vi "CRYSet Channel State.vi"(4 "New Channel Info":T1[](array[typedef]) {"Coupling" items=["Default"=-1, "RSE"=10083, "NRSE"=10078, "Differential"=10106, "Pseudodifferential"=12529]; "term config" items=["Default"=-1, "RSE"=10083, "NRSE"=10078, "Differential"=10106, "Pseudodifferential"=12529]; "Anti-aliasing Factor (%fs)" format="%.2f"}, 6 "Old Channel Info":T1[](array[typedef]) {"Coupling" items=["Default"=-1, "RSE"=10083, "NRSE"=10078, "Differential"=10106, "Pseudodifferential"=12529]; "term config" items=["Default"=-1, "RSE"=10083, "NRSE"=10078, "Differential"=10106, "Pseudodifferential"=12529]; "Anti-aliasing Factor (%fs)" format="%.2f"}, 9 "New Name In":string[][](array[string]), 10 "Old Name In":string[][](array[string]), 11 "Mode":enum16{"Load", "SaveAs", "Revert"}(ring)) -> (0 "Name Out":string[][](array[string]))   [LabVIEW 2013]
uses:
  Typedef Control/CRYHardware Channel Info.ctl
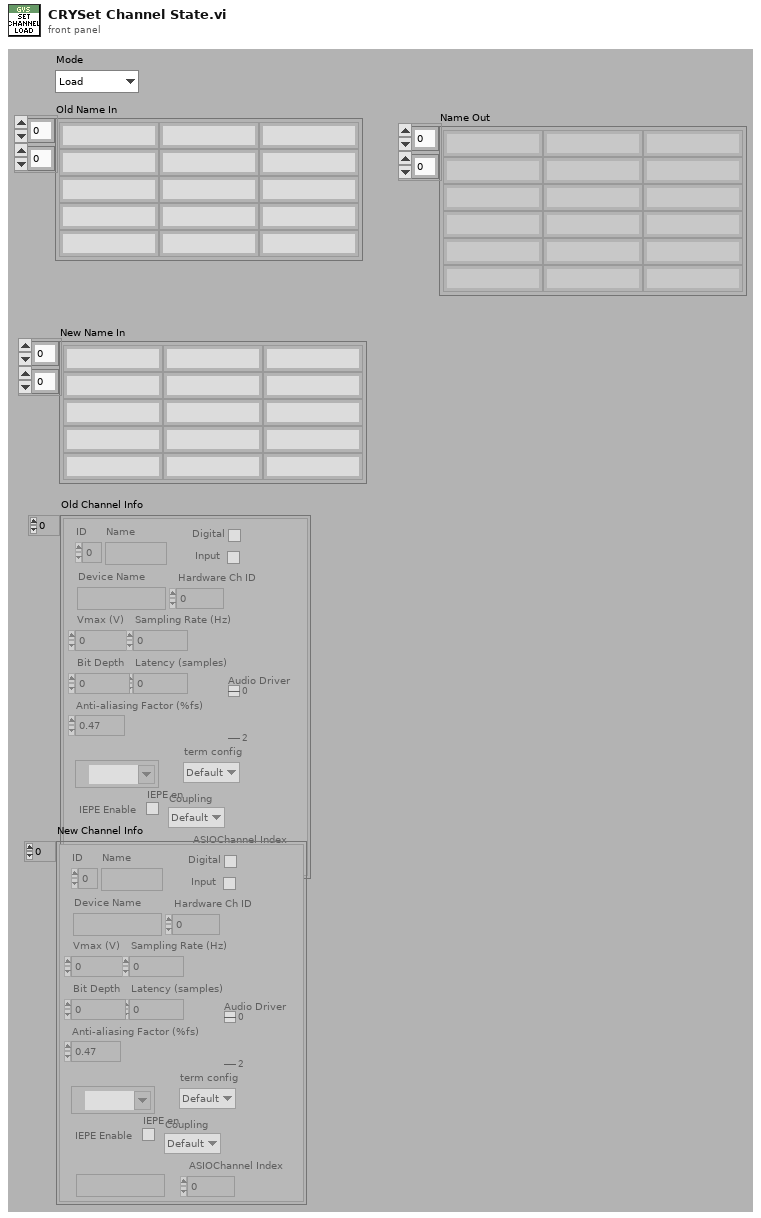
[diagram p1: front panel]
types:
  T1 = typedef "CRYHardware Channel Info.ctl" = cluster{"ID":i32, "Name":string, "Digital":bool, "Input":bool, "Device Name":string, "Hardware Ch ID":u8, "Vmax (V)":dbl, "Latency (samples)":dbl, "Sampling Rate (Hz)":u32, "Bit Depth":u32, "Anti-aliasing Factor (%fs)":sgl, "DAQmx Channel":tag, "term config":i32, "Coupling":i32, "IEPE en":bool, "ASIOChannel Name":string, "Audio Driver":u16, "ASIOChannel Index":u8}
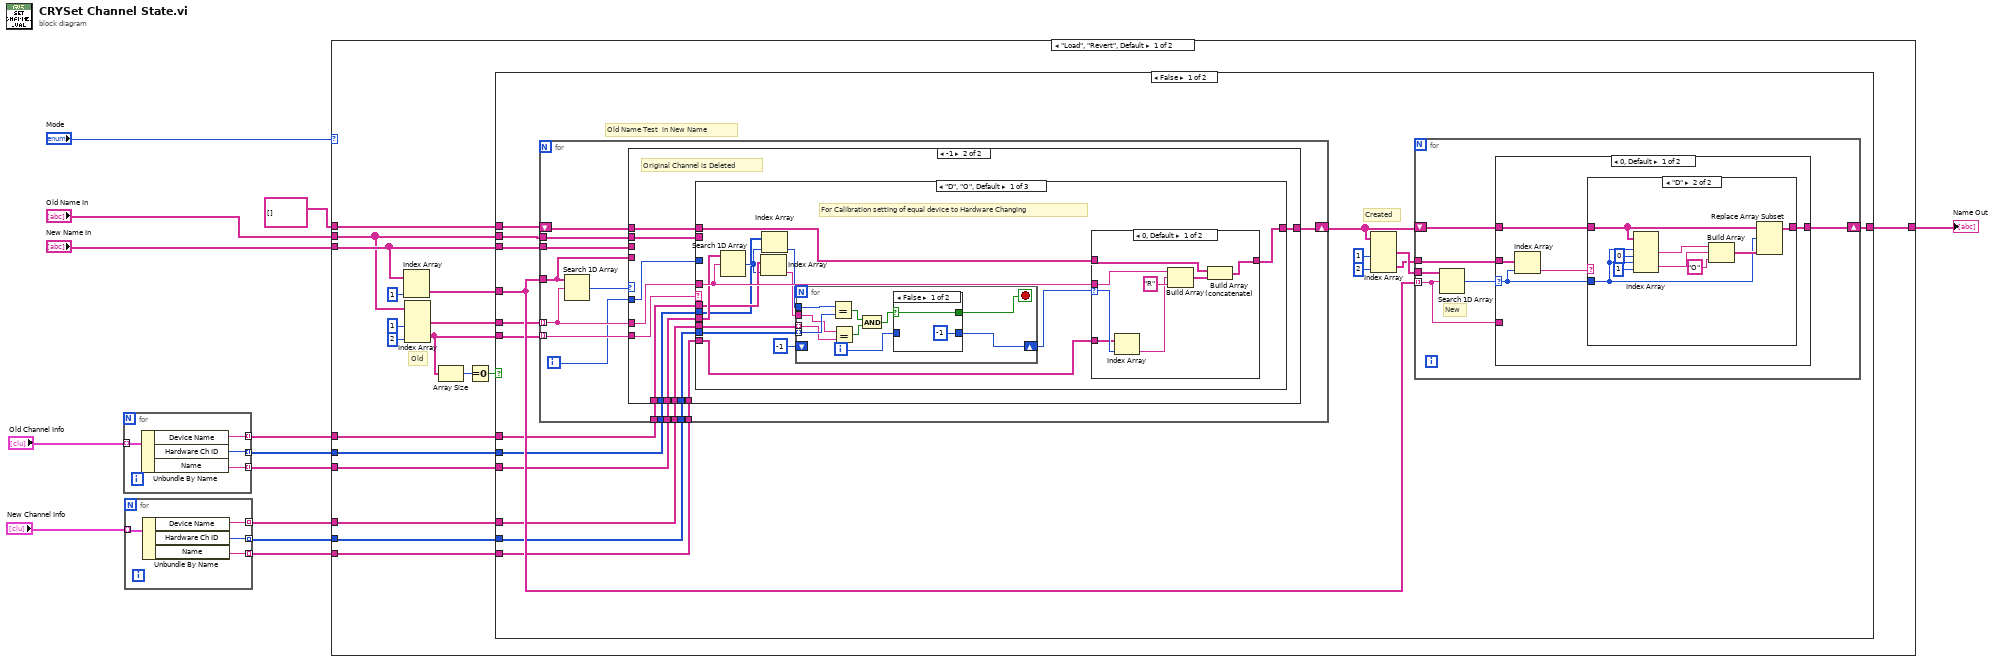
[diagram p0: block diagram]
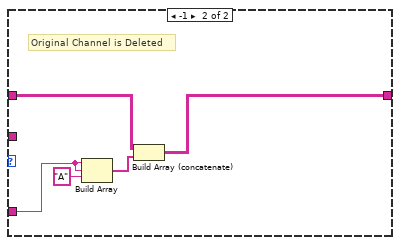
[diagram p3: hidden frame]
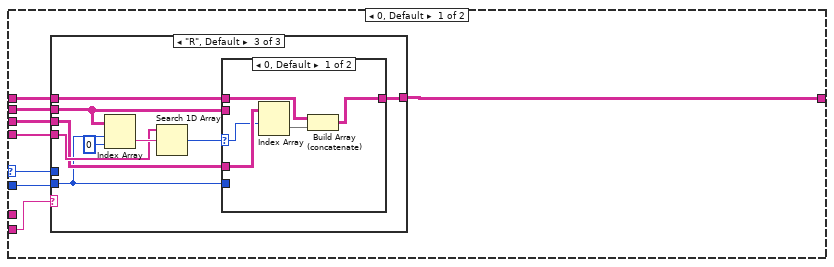
[diagram p4: hidden frame]
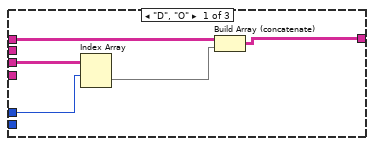
[diagram p5: hidden frame]
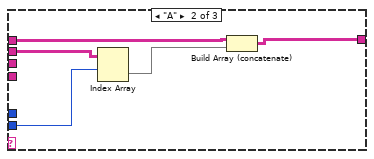
[diagram p6: hidden frame]
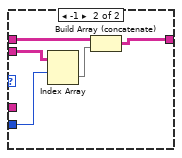
[diagram p7: hidden frame]
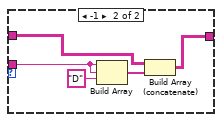
[diagram p9: hidden frame]
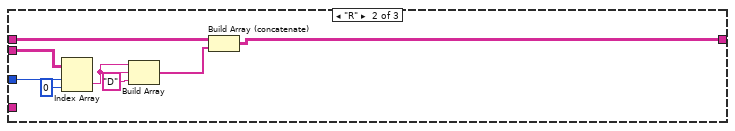
[diagram p10: hidden frame]
diagram:
  n1 = for {
    tunnel: "Old Channel Info" -> [w17] mode=indexing
    tunnel: [w16] -> w8 mode=indexing
    tunnel: [w15] -> w7 mode=indexing
    tunnel: [w14] -> w3 mode=indexing
    n2 = Unbundle By Name(w17) -> ("Device Name"=w16:string, "Hardware Ch ID"=w15:u8, "Name"=w14:string)
  }
  n3 = for {
    tunnel: "New Channel Info" -> [w21] mode=indexing
    tunnel: [w20] -> w5 mode=indexing
    tunnel: [w19] -> w4 mode=indexing
    tunnel: [w18] -> w2 mode=indexing
    n4 = Unbundle By Name(w21) -> ("Device Name"=w20:string, "Hardware Ch ID"=w19:u8, "Name"=w18:string)
  }
  n5 = case shown="\"Load\", \"Revert\", Default" "Mode" {
    tunnel: "New Name In" -> [w35 _]
    tunnel: [w36 w199] -> w12
    tunnel: string[][] [] ("Name Out") -> [w37 _]
    tunnel: "Old Name In" -> [w31 w199]
    tunnel: w8 -> [w27 _]
    tunnel: w7 -> [w26 _]
    tunnel: w5 -> [w25 _]
    tunnel: w4 -> [w24 _]
    tunnel: w3 -> [w23 _]
    tunnel: w2 -> [w22 _]
    frame "Load", "Revert", Default {
      # "Old"
      n6 = Index Array(array=w35, index (col)=1 ("disabled index (col)")) -> (element=w34:string[])  [unwired: 1 in]
      n7 = Index Array(array=w31, index (col) #1=1 ("disabled index (col)"), index (col) #2=2 ("index (col)")) -> (element #1=w33:string[], element #2=w30:string[])  [unwired: 2 in]
      n8 = Array Size(array=w30) -> (size(s)=w29:i32)
      n9 = Equal To 0?(x=w29) -> (x = 0?=w28:bool)
      n10 = case shown="False" w28 {
        tunnel: w37 -> [w57 _]
        tunnel: [w56 w198] -> w36
        tunnel: w35 -> [w55 w198]
        tunnel: w34 -> [w54 _]
        tunnel: w33 -> [w53 _]
        tunnel: w31 -> [w52 _]
        tunnel: w30 -> [w46 _]
        tunnel: w27 -> [w45 _]
        tunnel: w26 -> [w44 _]
        tunnel: w25 -> [w43 _]
        tunnel: w24 -> [w42 _]
        tunnel: w23 -> [w41 _]
        tunnel: w22 -> [w40 _]
        frame False {
          # "Created"
          # "Old Name Test  in New Name"
          n11 = for {
            tunnel: w54 -> [w90]
            tunnel: w53 -> [w97] mode=indexing
            shift-right: [w96] -> w51
            shift-left: w57 -> [w94]
            tunnel: w55 -> [w95]
            tunnel: w46 -> [w93] mode=indexing
            tunnel: w52 -> [w91]
            tunnel: w45 -> [w89]
            tunnel: w44 -> [w88]
            tunnel: w43 -> [w87]
            tunnel: w42 -> [w86]
            tunnel: w41 -> [w85]
            tunnel: w40 -> [w84]
            i -> [w92]
            n12 = Search 1D Array(1D array=w90, element=w97) -> (index of element=w98:i32)  [unwired: 1 in]
            n13 = case shown="-1" w98 {
              selector: w98 -> [w105 _]
              tunnel: w97 -> [_ w146]
              tunnel: [w99 w144] -> w96
              tunnel: w95 -> [w104 _]
              tunnel: w94 -> [w100 w145]
              tunnel: w93 -> [w106 w147]
              tunnel: w92 -> [w103 w142]
              tunnel: w91 -> [w102 w143]
              tunnel: w90 -> [w101 _]
              tunnel: w89 -> [_ w141]
              tunnel: w88 -> [_ w140]
              tunnel: w87 -> [_ w139]
              tunnel: w86 -> [_ w138]
              tunnel: w85 -> [_ w137]
              tunnel: w84 -> [_ w136]
              frame 0, Default {
                n14 = case shown="\"R\", Default" w106 {
                  tunnel: w105 -> [w111 _ _]
                  tunnel: w104 -> [w110 _ w121]
                  tunnel: w103 -> [_ w116 w117]
                  tunnel: w102 -> [_ w115 w118]
                  tunnel: w101 -> [_ _ w123]
                  tunnel: w100 -> [w109 w114 w120]
                  tunnel: [w107 w112 w119] -> w99
                  frame "D", "O" {
                    n15 = Index Array(array=w110, index (row)=w111) -> (element=w108:string[])  [unwired: 1 in]
                    n16 = Build Array (concatenate)(w109, w108) -> (w107:string[][])
                  }
                  frame "A" {
                    n17 = Index Array(array=w115, index (row)=w116) -> (element=w113:string[])  [unwired: 1 in]
                    n18 = Build Array (concatenate)(w114, w113) -> (w112:string[][])
                  }
                  frame "R", Default {
                    n19 = Index Array(array=w118, index (row)=w117, index (col)=0 ("disabled index (col)")) -> (element=w124:string)
                    n20 = Search 1D Array(1D array=w123, element=w124) -> (index of element=w122:i32)  [unwired: 1 in]
                    n21 = case shown="0, Default" w122 {
                      selector: w122 -> [w129 _]
                      tunnel: w121 -> [w130 _]
                      tunnel: w120 -> [w128 w134]
                      tunnel: [w126 w133] -> w119
                      tunnel: w118 -> [_ w135]
                      tunnel: w117 -> [_ w131]
                      frame 0, Default {
                        n22 = Index Array(array=w130, index (row)=w129) -> (element=w127:string[])  [unwired: 1 in]
                        n23 = Build Array (concatenate)(w128, w127) -> (w126:string[][])
                      }
                      frame -1 {
                        n24 = Index Array(array=w135, index (row)=w131) -> (element=w132:string[])  [unwired: 1 in]
                        n25 = Build Array (concatenate)(w134, w132) -> (w133:string[][])
                      }
                    }
                  }
                }
              }
              frame -1 {
                # "Original Channel is Deleted"
                n26 = case shown="\"D\", \"O\", Default" w147 {
                  tunnel: w146 -> [w159 _ _]
                  tunnel: w145 -> [w161 w195 w197]
                  tunnel: [w160 w196 w197] -> w144
                  tunnel: w143 -> [_ w194 _]
                  tunnel: w142 -> [_ w191 _]
                  tunnel: w141 -> [w157 _ _]
                  tunnel: w140 -> [w154 _ _]
                  tunnel: w139 -> [w153 _ _]
                  tunnel: w138 -> [w150 _ _]
                  tunnel: w137 -> [w158 _ _]
                  tunnel: w136 -> [w156 _ _]
                  frame "D", "O", Default {
                    # "For Calibration setting of equal device to Hardware Changing"
                    n27 = Search 1D Array(1D array=w158, element=w159) -> (index of element=w155:i32)  [unwired: 1 in]
                    n28 = Index Array(array=w157, index=w155) -> (element=w151:string)
                    n29 = Index Array(array=w154, index=w155) -> (element=w152:u8)
                    n30 = for {
                      tunnel: w153 -> [w168] mode=indexing
                      tunnel: w152 -> [w171]
                      tunnel: w151 -> [w169]
                      tunnel: w150 -> [w170] mode=indexing
                      shift-right: [w162] -> w149
                      shift-left: -1 -> [_]
                      i -> [w163]
                      stop <- w164 stop-if-true
                      n31 = Equal?(x=w171, y=w170) -> (x = y?=w166:bool)
                      n32 = Equal?(x=w169, y=w168) -> (x = y?=w167:bool)
                      n33 = And(x=w166, y=w167) -> (x .and. y?=w165:bool)
                      n34 = case shown="False" w165 {
                        selector: w165 -> [w172 w175]
                        tunnel: [w172 w175] -> w164
                        tunnel: w163 -> [_ w174]
                        tunnel: [-1 w174] -> w162
                        frame False {
                        }
                        frame True {
                        }
                      }
                    }
                    n35 = case shown="0, Default" w149 {
                      selector: w149 -> [w179 _]
                      tunnel: w161 -> [w181 w187]
                      tunnel: [w180 w186] -> w160
                      tunnel: w159 -> [w176 w184]
                      tunnel: w156 -> [w178 _]
                      frame 0, Default {
                        n36 = Index Array(array=w178, index=w179) -> (element=w177:string)
                        n37 = Build Array(w176, w177, "R" ("element")) -> (w182:string[])
                        n38 = Build Array (concatenate)(w181, w182) -> (w180:string[][])
                      }
                      frame -1 {
                        n39 = Build Array(w184, w184, "D" ("element")) -> (w185:string[])
                        n40 = Build Array (concatenate)(w187, w185) -> (w186:string[][])
                      }
                    }
                  }
                  frame "R" {
                    n41 = Index Array(array=w194, index (row)=w191, index (col)=0 ("disabled index (col)")) -> (element=w189:string)
                    n42 = Build Array(w189, w189, "D" ("Name")) -> (w192:string[])
                    n43 = Build Array (concatenate)(w195, w192) -> (w196:string[][])
                  }
                  frame "A" {
                  }
                }
              }
            }
          }
          n44 = Index Array(array=w51, index (col) #1=1 ("disabled index (col)"), index (col) #2=2 ("index (col)")) -> (element #1=w49:string[], element #2=w47:string[])  [unwired: 2 in]
          n45 = for {
            tunnel: w54 -> [w62] mode=indexing
            shift-right: [w61] -> w56
            shift-left: w51 -> [w60]
            tunnel: w49 -> [w59]
            tunnel: w47 -> [w58]
            # "New"
            n46 = Search 1D Array(1D array=w59, element=w62) -> (index of element=w63:i32)  [unwired: 1 in]
            n47 = case shown="0, Default" w63 {
              selector: w63 -> [w64 _]
              tunnel: w62 -> [_ w82]
              tunnel: [w65 w79] -> w61
              tunnel: w60 -> [w66 w81]
              tunnel: w58 -> [w68 _]
              frame 0, Default {
                n48 = Index Array(array=w68, index=w64) -> (element=w67:string)
                n49 = case shown="\"D\"" w67 {
                  tunnel: w66 -> [w69 w78]
                  tunnel: [w69 w77] -> w65
                  tunnel: w64 -> [_ w70]
                  frame "", Default {
                  }
                  frame "D" {
                    n50 = Index Array(array=w78, index (row) #1=w70, index (col) #1=0 ("disabled index (col)"), index (row) #2=w70, index (col) #2=1 ("disabled index (col)")) -> (element #1=w73:string, element #2=w72:string)
                    n51 = Build Array(w73, w72, "O" ("element")) -> (w74:string[])
                    n52 = Replace Array Subset(array=w78, new element=w74, index (row)=w70) -> (w77:string[][])  [unwired: 1 in]
                  }
                }
              }
              frame -1 {
                # "Original Channel is Deleted"
                n53 = Build Array(w82, w82, "A" ("element")) -> (w80:string[])
                n54 = Build Array (concatenate)(w81, w80) -> (w79:string[][])
              }
            }
          }
        }
        frame True {
          # "When First Loading."
        }
      }
    }
    frame "SaveAs" {
      # "????????????"
    }
  }
  "Name Out" <- w12
